vi "SwissSPAD Live_Settings Timeout.vi"(8 "Error In":errorcluster, 11 "Settings Control Refnums":T1) -> (0 "Error Out":errorcluster)   [LabVIEW 2021]
uses:
  SwissSPAD Live_SS3 DAQ Parameters.ctl
  SwissSPAD Live_SS3 Gate Definition.ctl
  SS3 Gate Width Definition Mode.ctl
  SwissSPAD Live_SS3 Displayed Image v2.ctl
  SwissSPAD Live_Settings List.ctl
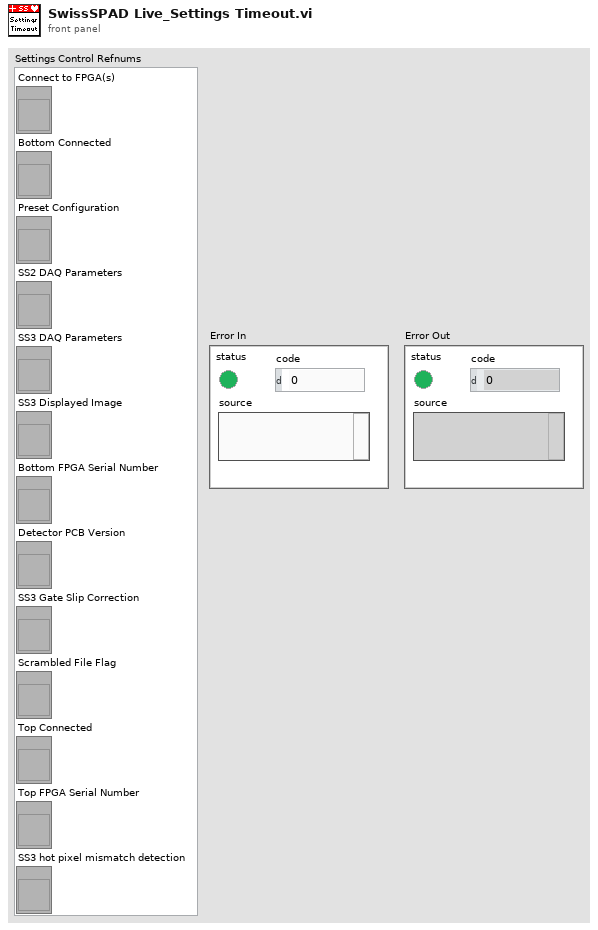
[diagram p1: front panel]
types:
  T1 = cluster{"Connect to FPGA(s)":refnum<vi>, "Bottom Connected":refnum<vi>, "Preset Configuration":refnum<vi>, "SS2 DAQ Parameters":refnum<vi>, "SS3 DAQ Parameters":refnum<vi>, "SS3 Displayed Image":refnum<vi>, "Bottom FPGA Serial Number":refnum<vi>, "Detector PCB Version":refnum<vi>, "SS3 Gate Slip Correction":refnum<vi>, "Scrambled File Flag":refnum<vi>, "Top Connected":refnum<vi>, "Top FPGA Serial Number":refnum<vi>, "SS3 hot pixel mismatch detection":refnum<vi>}
  T2 = typedef "SwissSPAD Live_Settings List.ctl" = enum16{"FPGA:Bottom Half", "FPGA:Top Half", "FPGA:Bottom Bitfile Path", "FPGA:Top Bitfile Path", "FPGA:Bottom Bitstream Version", "FPGA:Top Bitstream Version", "FPGA:Auto Reset FPGA", "FPGA:Bottom FPGA Serial Number", "FPGA:Top FPGA Serial Number", "FPGA:Detector PCB Version", "Acquisition Parameters:Microlens", "Acquisition Parameters:SS2 DAQ Parameters", "Acquisition Parameters:Gate Configuration Array", "Acquisition Parameters:SS3 DAQ Parameters", "Acquisition Parameters:Buffer Size (# 8-bit Gates)", "File Information:File Information", "File Information:# Datasets in Series", "File Information:Scrambled File Flag", "File Information:SS3 Gate Slip Correction", "File Information:SS3 Hot Pixel Mismatch Detection", "File Information:Delay between Datasets", "File Information:Save Sum of All Gates Preview", "Image Parameters:Image ROI Information", "Image Parameters:Image Binning Options", "Image Parameters:SS3 Displayed Image", "Image Parameters:Image Display Options", "Image Parameters:Use Histogram Cursors", "Image Parameter:FPGA Data to Display", "UI Settings:Histogram Bins Number", "UI Settings:Histogram Bin Size", "UI Settings:Use Image Display Options", "UI Settings:Verbose Settings", "UI Settings:Verbose Saving"}
  T3 = typedef "SwissSPAD Live_Internal Variables.ctl" = cluster{"okCFrontPanelDevices Refnum":refnum<k24>, "Bottom Device Refnum":refnum<k24>, "Display Image":T4, "# Live Images":i32, "relative s":dbl, "# Image Sets":i32, "Message":string, "Current Image Set":i32, "# Datasets in Series":i32, "Current Dataset":i32, "Live Mode":bool, "Recording Mode":bool, "Record Button":refnum<vi>, "\nLive Button":refnum<vi>, "SwissSPAD Live Gate Image Data Q Name":string, "Discard First Image":bool, "Image Information":T5, "Image Binning Options":T6, "Bottom FPGA Serial Number":string, "Detector PCB Version":T7, "# Acquisitions":u32, "10 bits":bool, "Top FPGA Serial Number":string, "Top Device Refnum":refnum<k24>, "okCFrontPanel Refnum":refnum<k24>}
  T4 = typedef "IMAQ Image.ctl" = refnum<image>
  T5 = typedef "SwissSPAD Live_Image ROI Information.ctl" = cluster{"Save ROI Only":bool, "Left":u16, "Top":u16, "Right":u16, "Bottom":u16, "Use Current ROI":bool}
  T6 = typedef "Image Binning Options.ctl" = cluster{"Use Image Binning":bool, "X Bin":i32, "Y Bin":i32}
  T7 = typedef "SwissSPAD Live_SSx PCB Version.ctl" = enum16{"unknown", "SS2 PCB1", "SS2 PCB2", "SS3 PCB1"}
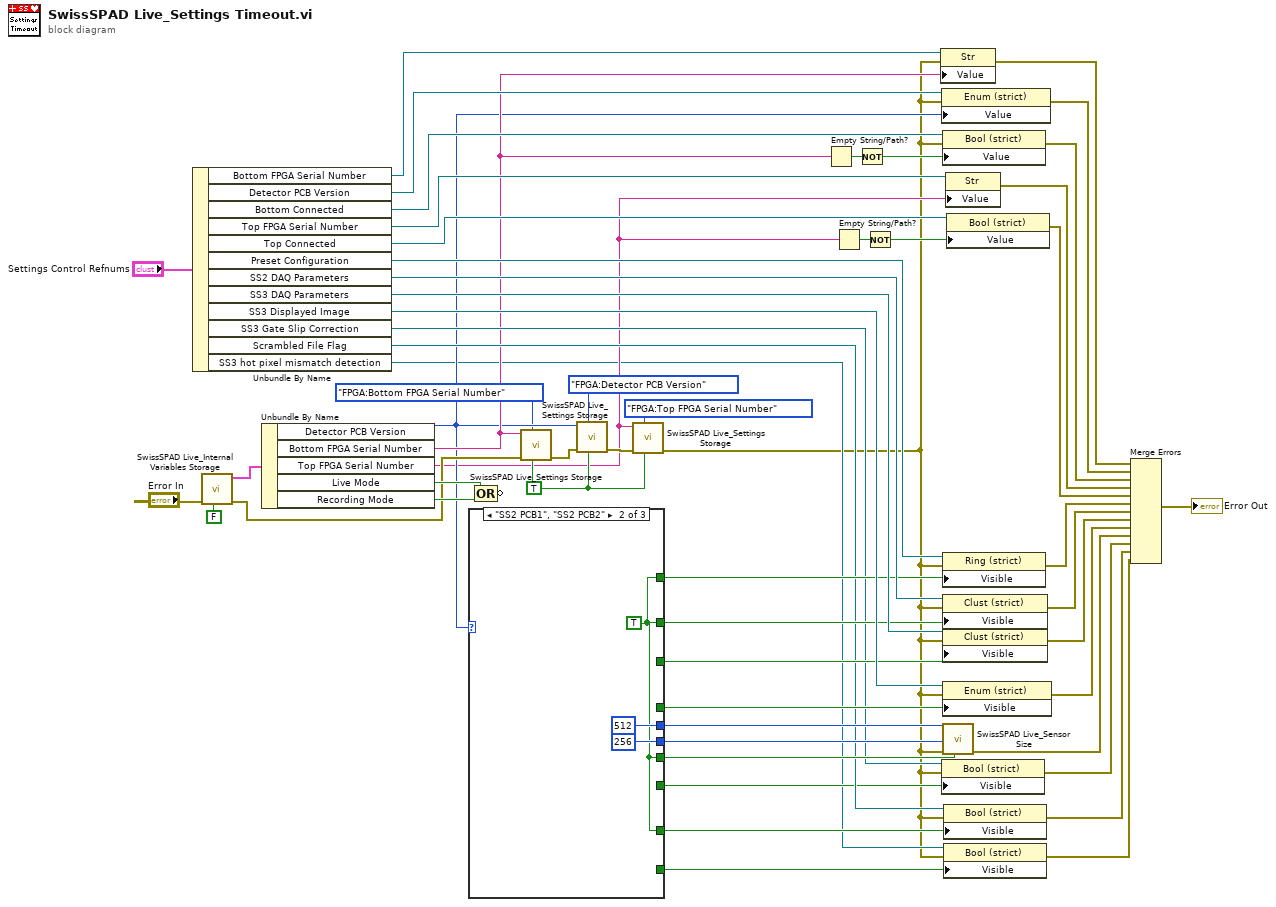
[diagram p0: block diagram]
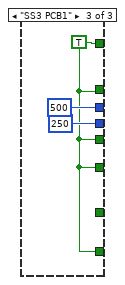
[diagram p3: hidden frame]
diagram:
  w21 = TRUE ("Set/Get(F)")
  n1 = Unbundle By Name("Settings Control Refnums") -> ("Bottom FPGA Serial Number"=w32:refnum<vi>, "Detector PCB Version"=w31:refnum<vi>, "Bottom Connected"=w49:refnum<vi>, "Top FPGA Serial Number"=w19:refnum<vi>, "Top Connected"=w16:refnum<vi>, "Preset Configuration"=w50:refnum<vi>, "SS2 DAQ Parameters"=w52:refnum<vi>, "SS3 DAQ Parameters"=w55:refnum<vi>, "SS3 Displayed Image"=w56:refnum<vi>, "SS3 Gate Slip Correction"=w28:refnum<vi>, "Scrambled File Flag"=w26:refnum<vi>, "SS3 hot pixel mismatch detection"=w5:refnum<vi>)
  n2 = call "SwissSPAD Live_Internal Variables Storage.vi"("Set/Get(F)"=FALSE, "Error In"="Error In") -> ("Error Out"=w20:errorcluster, "SwissSPAD Live Internal Variables"=w41:T3)  [unwired: 8 in]
  n3 = Unbundle By Name(w41) -> ("Detector PCB Version"=w7:T7, "Bottom FPGA Serial Number"=w8:string, "Top FPGA Serial Number"=w6:string, "Live Mode"=w43:bool, "Recording Mode"=w44:bool)
  n4 = case shown="\"SS2 PCB1\", \"SS2 PCB2\"" w7 {
    tunnel: [_ w58 _] -> w51
    tunnel: [_ w58 _] -> w53
    tunnel: [_ _ w61] -> w54
    tunnel: [_ _ w61] -> w57
    tunnel: [_ 512 ("X size") 500 ("X size")] -> w45
    tunnel: [_ 256 ("Y size") 250 ("Y size")] -> w46
    tunnel: [_ w58 w61] -> w47
    tunnel: [_ _ w61] -> w24
    tunnel: [_ w58 _] -> w23
    tunnel: [_ _ w61] -> w3
    frame "unknown", Default {
    }
    frame "SS2 PCB1", "SS2 PCB2" {
      w58 = TRUE ("Visible")
    }
    frame "SS3 PCB1" {
      w61 = TRUE ("Visible")
    }
  }
  n5 = Compound Arithmetic op=OR(w43, w44) -> ()  [unwired: 1 out]
  n6 = call "SwissSPAD Live_Settings Storage.vi"("Set/Get(F)"=w21, "Settings List"=SwissSPAD_Live_Settings_List."FPGA:Bottom FPGA Serial Number", "Error In"=w20, "Variant Data in"=w8) -> ("Error Out"=w40:errorcluster)  [unwired: 6 in, 1 out]
  n7 = call "SwissSPAD Live_Settings Storage.vi"("Set/Get(F)"=w21, "Settings List"=SwissSPAD_Live_Settings_List."FPGA:Detector PCB Version", "Error In"=w40, "Variant Data in"=w7) -> ("Error Out"=w22:errorcluster)  [unwired: 6 in, 1 out]
  n8 = call "SwissSPAD Live_Settings Storage.vi"("Set/Get(F)"=w21, "Settings List"=SwissSPAD_Live_Settings_List."FPGA:Top FPGA Serial Number", "Error In"=w22, "Variant Data in"=w6) -> ("Error Out"=w4:errorcluster)  [unwired: 6 in, 1 out]
  n9 = Empty String/Path?(string/path=w8) -> (empty?=w18:bool)
  n10 = Empty String/Path?(string/path=w6) -> (empty?=w15:bool)
  n11 = Not(x=w18) -> (.not. x?=w17:bool)
  n12 = Not(x=w15) -> (.not. x?=w14:bool)
  n13 = property class="Str"(reference=w32, error in=w4, "Value"=w8) -> (error out=w30:errorcluster)  [unwired: 1 out]
  n14 = property class="Enum (strict)"(reference=w31, error in=w4, "Value"=w7) -> (error out=w29:errorcluster)  [unwired: 1 out]
  n15 = property class="Bool (strict)"(reference=w28, error in=w4, "Visible"=w24) -> (error out=w27:errorcluster)  [unwired: 1 out]
  n16 = property class="Bool (strict)"(reference=w49, error in=w4, "Value"=w17) -> (error out=w13:errorcluster)  [unwired: 1 out]
  n17 = property class="Ring (strict)"(reference=w50, error in=w4, "Visible"=w51) -> (error out=w39:errorcluster)  [unwired: 1 out]
  n18 = property class="Clust (strict)"(reference=w52, error in=w4, "Visible"=w53) -> (error out=w38:errorcluster)  [unwired: 1 out]
  n19 = property class="Clust (strict)"(reference=w55, error in=w4, "Visible"=w54) -> (error out=w37:errorcluster)  [unwired: 1 out]
  n20 = property class="Enum (strict)"(reference=w56, error in=w4, "Visible"=w57) -> (error out=w36:errorcluster)  [unwired: 1 out]
  n21 = call "SwissSPAD Live_Sensor Size.vi"("Set/Get(F)"=w47, "Error In"=w4, "Y size"=w46, "X size"=w45) -> ("Error Out"=w35:errorcluster)  [unwired: 5 in, 2 out]
  n22 = property class="Bool (strict)"(reference=w26, error in=w4, "Visible"=w23) -> (error out=w25:errorcluster)  [unwired: 1 out]
  n23 = property class="Bool (strict)"(reference=w5, error in=w4, "Visible"=w3) -> (error out=w2:errorcluster)  [unwired: 1 out]
  n24 = property class="Str"(reference=w19, "Value"=w6) -> (error out=w12:errorcluster)  [unwired: 1 in, 1 out]
  n25 = property class="Bool (strict)"(reference=w16, "Value"=w14) -> (error out=w11:errorcluster)  [unwired: 1 in, 1 out]
  n26 = Merge Errors(w30, w29, w13, w12, w11, w39, w38, w37, w36, w35, w27, w25, w2) -> (→"Error Out":errorcluster)
